vi "ScaleCIC_5.vi"(8 "input valid":bool=TRUE, 11 "x":fxp<+/-,32,32>) -> (0 "valid out":bool, 3 "Data out":fxp<+/-,16,14>)   [LabVIEW 2013]
uses:
  <vilib>/rvi/FXPMathLib/FxpInterpret/XNode/nifxpmath_Interpret.xnode
  <vilib>/rvi/FXPMathLib/FxpMul/XNode/nifxpmath_Multiplier.xnode
  <vilib>/rvi/FXPMathLib/sim/FxpSim.dll
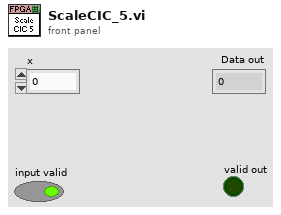
[diagram p1: front panel]
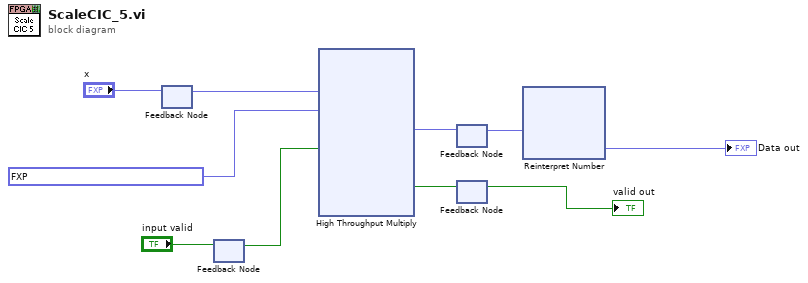
[diagram p0: block diagram]
diagram:
  n1 = feedback #1() -> (w3:fxp<+/-,32,32>)  [unwired: 1 in]
  n2 = feedback-in #1("x") -> ()
  n3 = feedback #2() -> (w1:bool)  [unwired: 1 in]
  n4 = feedback-in #2("input valid") -> ()
  n5 = xnode ("High Throughput Multiply")("x"=w3, "y"=fxp<+/-,32,1> 0.001600000075995922, "input valid"=w1) -> ("x*y"=w8:fxp<+/-,16,16>, "output valid"=w6:bool)  [unwired: 1 in, 1 out]
  n6 = feedback #3() -> (w7:fxp<+/-,16,16>)  [unwired: 1 in]
  n7 = feedback-in #3(w8) -> ()
  n8 = feedback #4() -> (→"valid out":bool)  [unwired: 1 in]
  n9 = feedback-in #4(w6) -> ()
  n10 = xnode "Reinterpret Number"("x"=w7) -> ("y"=→"Data out":fxp<+/-,16,14>)
